vi "Update Global Vars.vi"(8 "Error In":errorcluster, 10 "Nufern Digital Timing Control 2":refnum<vi>, 11 "Scanning Parameters":refnum<vi>) -> (0 "Error Out":errorcluster)   [LabVIEW 2015]
uses:
  Classes/Galvo/Scanning Cluster.ctl
  Scan Parameters Global Variable.vi
  Classes/Nufern/Nufern Digital Control Global.vi
  Classes/Galvo/Galvo.lvclass
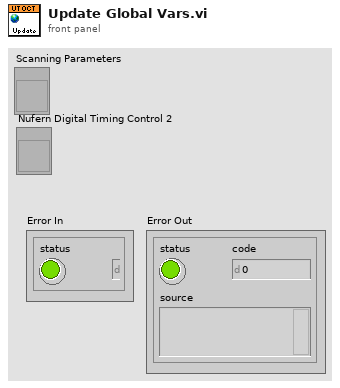
[diagram p1: front panel]
types:
  T1 = typedef "Nufern Digital Timing Control.ctl" = cluster{"Fire":bool, "Start A-Scan":u32, "Stop A-Scan":u32, "Reps per Fire":i32, "B-Scan Spacing":i32}
  T2 = typedef "Galvo.lvclass/Scanning Cluster.ctl" = cluster{"Fast Axis Offset":sgl, "Slow Axis Offset":sgl, "Slow Axis Amp":sgl, "Fast Axis Amp":sgl, "Scan Pattern":enum16{"Raster", "Triangle Raster", "Sinusoid Raster"}}
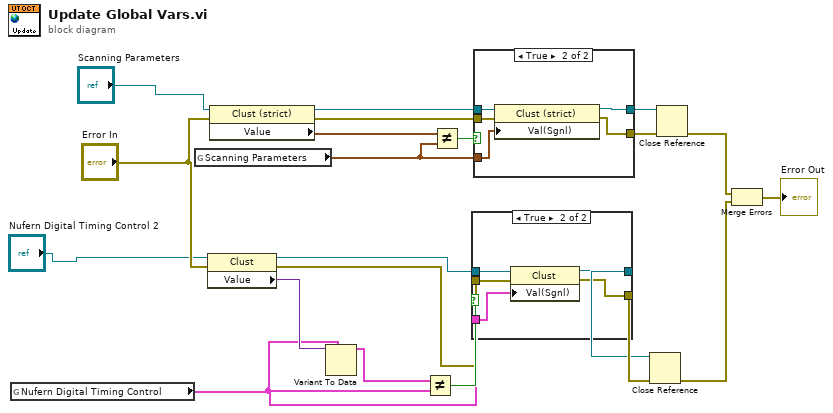
[diagram p0: block diagram]
diagram:
  n1 = global read "Nufern Digital Control Global.vi" "Nufern Digital Timing Control"() -> (w2:T1)
  n2 = global read "Scan Parameters Global Variable.vi" "Scanning Parameters"() -> (w20:T2)
  n3 = property class="Clust"(reference="Nufern Digital Timing Control 2", error in="Error In") -> (reference out=w12:refnum<vi>, error out=w11:errorcluster, "Value"=w3:variant)
  n4 = property class="Clust (strict)"(reference="Scanning Parameters", error in="Error In") -> (reference out=w19:refnum<vi>, error out=w16:errorcluster, "Value"=w17:T2)
  n5 = Variant To Data(type=w2, Variant=w3) -> (data=w1:T1)  [unwired: 1 in, 1 out]
  n6 = Not Equal?(x=w1, y=w2) -> (x != y?=w13:bool)
  n7 = Not Equal?(x=w17, y=w20) -> (x != y?=w18:bool)
  n8 = case shown="True" w13 {
    tunnel: w12 -> [w23 w28]
    tunnel: w2 -> [_ w27]
    tunnel: [w23 w26] -> w7
    tunnel: w11 -> [w22 w25]
    tunnel: [w22 w24] -> w8
    frame False {
    }
    frame True {
      n9 = property class="Clust"(reference=w28, error in=w25, "Val(Sgnl)"=w27) -> (reference out=w26:refnum<vi>, error out=w24:errorcluster)
    }
  }
  n10 = case shown="True" w18 {
    tunnel: w19 -> [w30 w35]
    tunnel: w20 -> [_ w34]
    tunnel: [w30 w33] -> w21
    tunnel: w16 -> [w29 w32]
    tunnel: [w29 w31] -> w15
    frame False {
    }
    frame True {
      n11 = property class="Clust (strict)"(reference=w35, error in=w32, "Val(Sgnl)"=w34) -> (reference out=w33:refnum<vi>, error out=w31:errorcluster)
    }
  }
  n12 = Close Reference(reference=w7, error in (no error)=w8) -> (error out=w6:errorcluster)
  n13 = Close Reference(reference=w21, error in (no error)=w15) -> (error out=w9:errorcluster)
  n14 = Merge Errors(w9, w6) -> (→"Error Out":errorcluster)
